vi "Drive_Globals.vi"() -> ()   [LabVIEW 2019]
uses:
  Drive_Cluster.ctl
  Drive_States.ctl
  Utility_VIs/Basic_Motor_Modes.ctl
panel:
  in  "Motor_Mode":T1
  in  "Right Motor Output":dbl
  in  "Left Motor Output":dbl
  in  "Drive_IMU":string="Drive_IMU"
  in  "Drive_Left_Master":string="Drive_Left_Master"
  in  "Drive_Left_Slave":string="Drive_Left_Slave"
  in  "Drive_Right_Slave":string="Drive_Right_Slave"
  in  "Drive_Right_Master":string="Drive_Right_Master"
  in  "Drive_Execute_Notifier":refnum<notifier>
  in  "Drive_Set_Notifier":refnum<notifier>
  in  "Drive_Execute_Ref":string="Drive_Execute_Ref"
  in  "Drive_Set_Ref":string="Drive_Set_Ref"
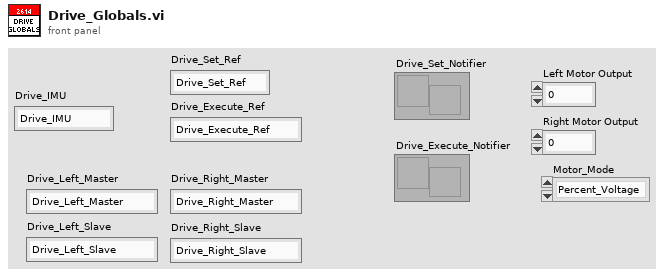
[diagram p1: front panel]
types:
  T1 = typedef "Basic_Motor_Modes.ctl" = enum16{"Percent_Voltage", "Speed_Control", "Position_Control", "Current"}
diagram:
